vi "Throw Post Step Runtime Error.vi"(0 "Error Message":string, 11 "error in":errorcluster) -> (15 "error out":errorcluster)   [LabVIEW 2023, in "RFCalAndFixtureCharact.Common.lvlib"]
uses:
  RFCalAndFixtureCharact.Common.lvlib
  Global Post Step Runtime Error ID.vi
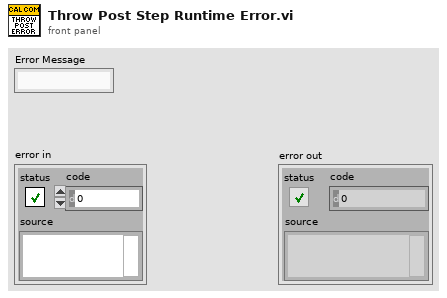
[diagram p1: front panel]
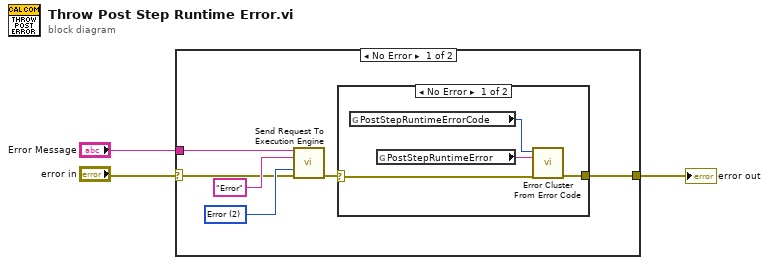
[diagram p0: block diagram]
diagram:
  n1 = case shown="No Error" "error in" {
    selector: "error in" -> [w6 w15]
    tunnel: [w5 w15] -> w3
    tunnel: "Error Message" -> [w7 _]
    frame No Error {
      w8 = 2 items=["Info", "Warning", "Error", "Action"] ("Message Type")
      n2 = call "Send Request To Execution Engine.vi"("Request Message"=w7, "Request Header"="Error", "Request Content Type"=w8, "error in (no error)"=w6) -> ("error out"=w4:errorcluster)  [unwired: 10 in, 1 out]
      n3 = case shown="No Error" w4 {
        selector: w4 -> [w10 w14]
        tunnel: [w11 w14] -> w5
        frame No Error {
          n4 = global read "Global Post Step Runtime Error ID.vi" "PostStepRuntimeErrorCode"() -> (w12:i32)
          n5 = global read "Global Post Step Runtime Error ID.vi" "PostStepRuntimeError"() -> (w13:string)
          n6 = call <vilib>:"Error Cluster From Error Code.vi"("error in (no error)"=w10, "error message (\"\")"=w13, "error code (0)"=w12) -> ("error out"=w11:errorcluster)  [unwired: 6 in]
        }
        frame Error {
        }
      }
    }
    frame Error {
    }
  }
  "error out" <- w3
